vi "LV to ITX Retrieve Equation.vi"(0 "File or Folder Path":path=path "\\\\TILES\\Data/SA02777G.graphene.20150414/12 - sweep B +-2T, step Vsg", 5 "offset":i32, 7 "length":i32=10, 9 "index":T1={"a"=3, "b"=5, "c"=7, "d"=9, "f"=2, "N1"=2, "N2"=0, "N3"=0, "N4"=0, "g"=2}) -> (4 "y1 vs g":cluster{dbl[], dbl[]}[](graph), 6 "y2 vs g":cluster{dbl[], dbl[]}[](graph), 8 "2D":dbl[][](graph), 10 "N":cluster{"N1":dbl, "N2":dbl, "N3":dbl, "N4":dbl}={"N1"=0.0, "N2"=3512286493.887331, "N3"=3512286493.887331, "N4"=3512286493.887331} {"N4" format="%#_6p"; "N3" format="%#_6p"; "N2" format="%#_6p"; "N1" format="%#_6p"}, 14 "Comments":string="sweep Vsg (22): 750mV to -500mV 50mV steps\r\n\r\n\r\n\r\n\r\n\r\n\r\n\r\n\r\n\r\n\r\n\r\n\r\n\r\n\r\nB=0T to 2T to -2T to 0T, 0.0104 A/s\r\n\r\n\r\n\r\n\r\n\r\n\r\n\r\n\r\n\r\n\r\n\r\n\r\n\r\n\r\n\r\n\r\n\r\n\r\n\r\n\r\n\r\n\r\n\r\n\r\n\r\n\r\n\r\n\r\n\r\nlockin\r\n\r\n\r\n\r\n\r\n\r\n\r\n\r\n\r\n\r\n\r\n\r\n\r\n\r\n\r\n0: 1\r\n\r\n\r\n\r\n\r\n\r\n\r\n\r\n\r\n\r\n\r\n\r\n\r\n\r\n\r\n1: 3\r\n\r\n\r\n\r\n\r\n\r\n\r\n\r\n\r\n\r\n\r\n\r\n\r\n\r\n\r\n2: 4, current\r\n\r\n\r\n\r\n\r\n\r\n\r\n\r\n\r\n\r\n\r\n\r\n\r\n\r\n\r\n3: 5\r\n\r\n\r\n\r\n\r\n\r\n\r\n\r\n\r\n\r\n\r\n\r\n\r\n\r\n\r\n4: 27\r\n\r\n\r\n\r\n\r\n\r\n\r\n\r\n\r\n\r\n\r\n\r\n\r\n\r\n\r\n5: 28, current, 8mV AC\r\n\r\n\r\n\r\n\r\n\r\n\r\n\r\n\r\n\r\n\r\n\r\n\r\n\r\n\r\nappliedVsg= 0.300000\r\n\r\n\r\n\r\n\r\n\r\n\r\n\r\n\r\n\r\n\r\n\r\n\r\n\r\n\r\n")   [LabVIEW 2016, in "LVtoITX.lvclass"]
uses:
  LVtoITX.lvclass
  <vilib>/Utility/miscctls.llb/LVOffsetAndMultiplierTypeDef.ctl
  <vilib>/gmath/NI_Gmath.lvlib
panel:
  in  "2D graph:\non = y1\noff = y2":bool=TRUE
  in  "DAT header length":i32=11
  in  "data length":i32=2500
  in  "data index":i32=1400
  in  "string formula":bool caption="string formula = ON (slow, easy prototyping)\nblock diagram formula = OFF (fast, must edit block diagram to change))"
  in  "Enum":enum16{"ITX", "ITX w/ 2D", "DAT"}(ring)=enum."DAT"
  in  "formula (parameters: a,b,c,d,f)":string="y1 = (a-b)/c;\ny2 = (b-d)/c;"
  in  "D  is time?":bool
  in  "B is time?":bool
  out "time":string[][](table)=[["4/18/2015", "12:40 PM"], ["4/18/2015", "5:05 PM"], ["4/18/2015", "10:04 PM"], ["4/18/2015", "11:37 PM"], ["4/19/2015", "1:07 AM"], ["4/19/2015", "2:37 AM"], ["4/19/2015", "4:07 AM"], ["4/19/2015", "5:37 AM"], ["4/19/2015", "7:08 AM"], ["4/19/2015", "8:38 AM"]]
  in  "Use Folder Index File?":bool
  in  "Generate Folder Index File?":bool
  in  "Ez name":string="Ez name"
  in  "Ey name":string="Ey name"
  in  "Ex name":string="Ex name"
  in  "C y name":string="C y name"
  in  "D x name":string="D x name"
  in  "A y name":string="A y name"
  in  "B x name":string="B x name"
  out "Index, Wavenames":string[][](table)=[["0", "time"], ["1", "temp"], ["2", "Bfield"], ["3", "X0"], ["4", "Y0"], ["5", "X1"], ["6", "Y1"], ["7", "X2"], ["8", "Y2"], ["9", "X3"], ["10", "Y3"], ["11", "X4"], ["12", "Y4"], ["13", "X5"], ["", "Y5"]]
  in  "recolor traces?":bool=TRUE
  in  "Ex":T2={"Offset"=0.0, "Multiplier"=1.0}
  in  "Ey":T2={"Offset"=0.0, "Multiplier"=1.0}
  out "Path":path=path "\\\\TILES\\Data/SA02777G.graphene.20150414/12 - sweep B +-2T, step Vsg/SA02777G.graphene.20150414.000009.dat"
  out "counter":i32=9
  in  "pattern":string="*.dat"
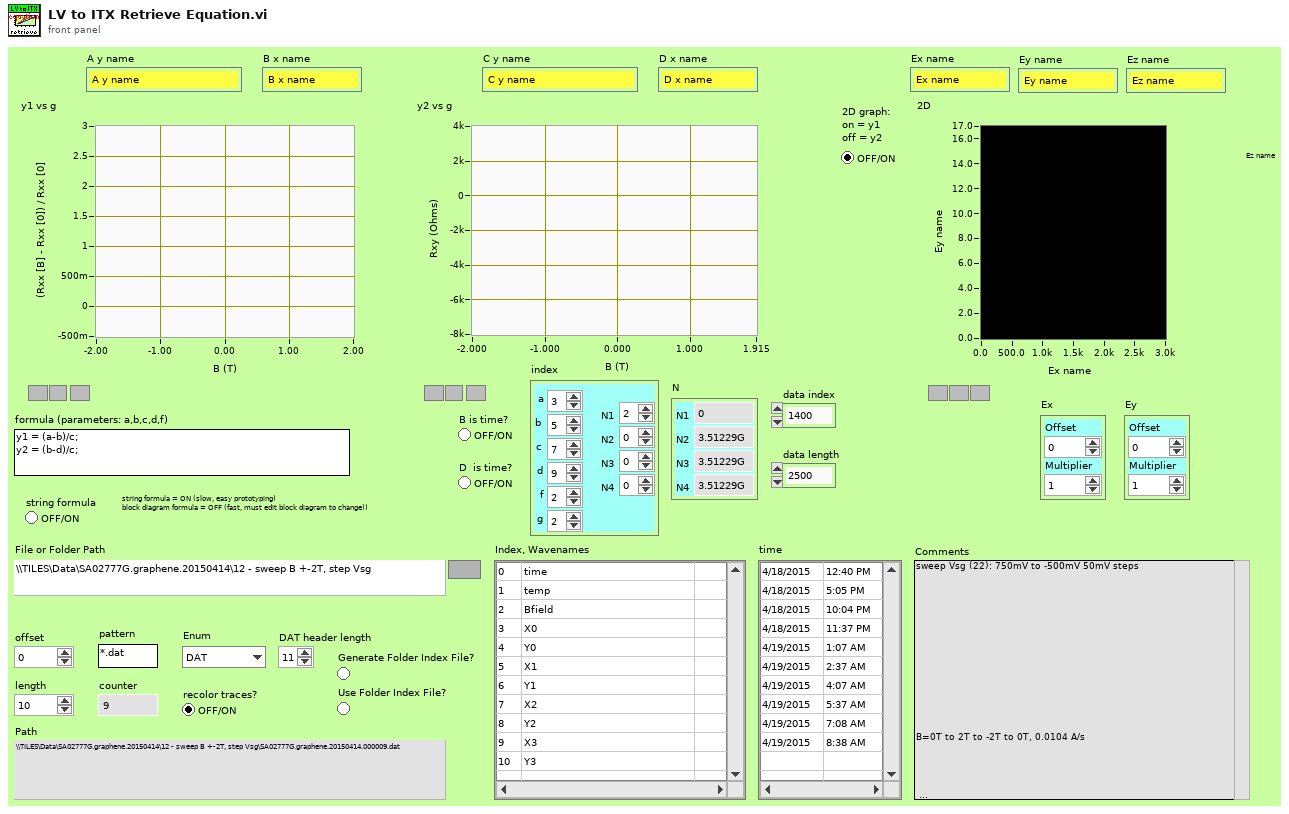
[diagram p1: front panel]
types:
  T1 = cluster{"a":i32, "b":i32, "c":i32, "d":i32, "f":i32, "N1":i32, "N2":i32, "N3":i32, "N4":i32, "g":i32}
  T2 = typedef "LVOffsetAndMultiplierTypeDef.ctl" = cluster{"Offset":dbl, "Multiplier":dbl}
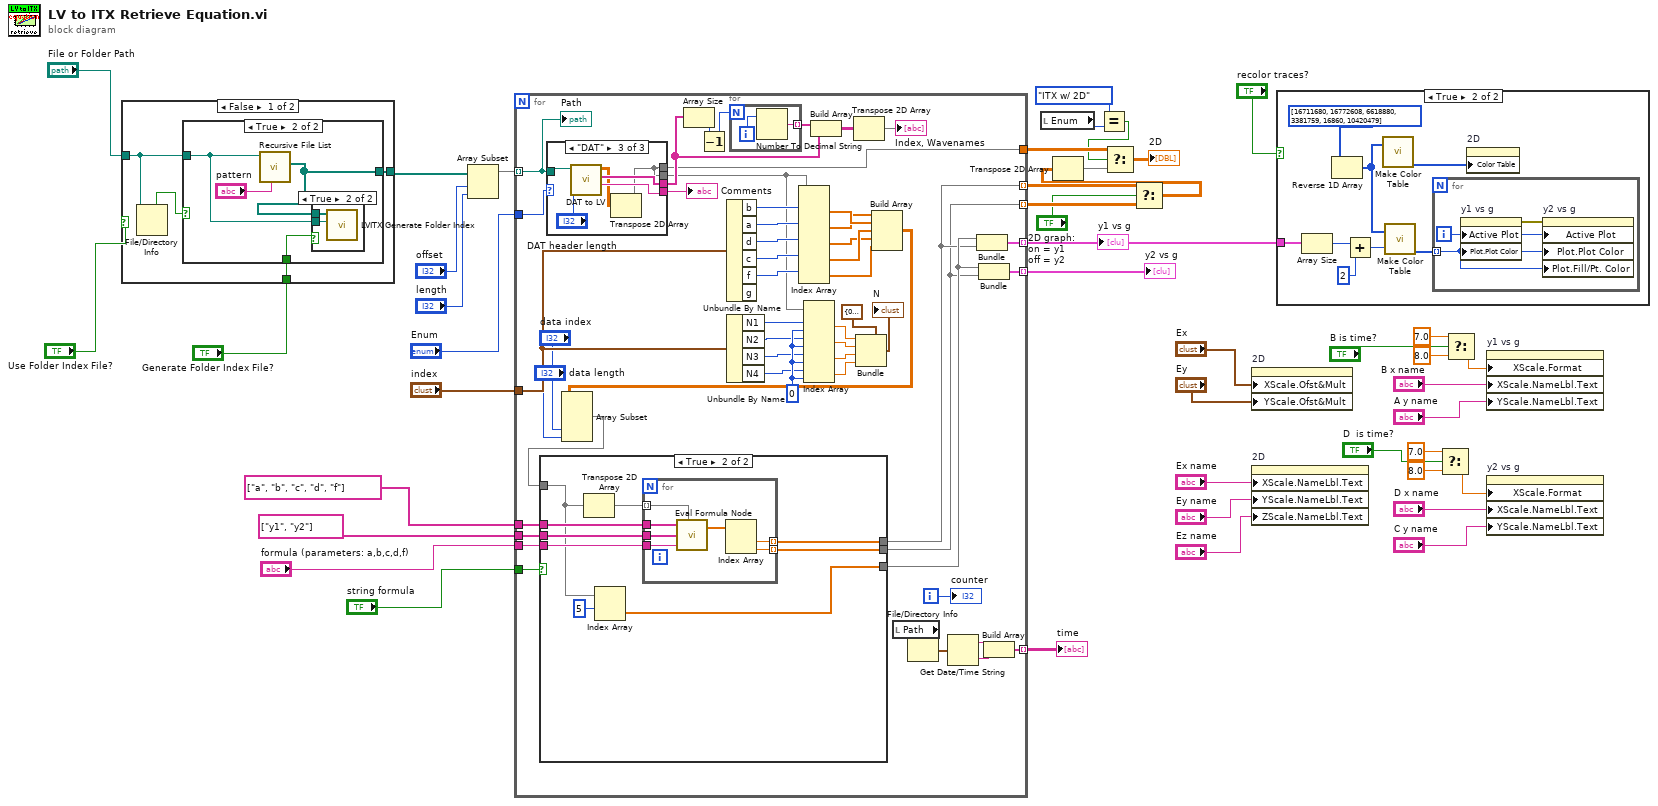
[diagram p0: block diagram]
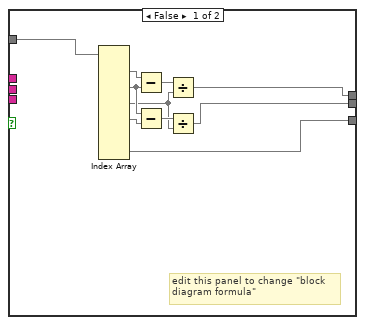
[diagram p3: hidden frame]
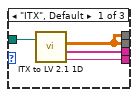
[diagram p4: hidden frame]
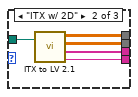
[diagram p5: hidden frame]
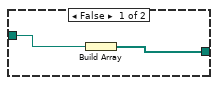
[diagram p6: hidden frame]
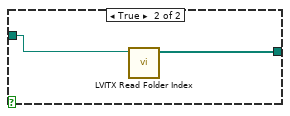
[diagram p8: hidden frame]
diagram:
  n1 = case shown="False" "Use Folder Index File?" {
    tunnel: [w46 w57] -> w42
    tunnel: "File or Folder Path" -> [w48 w58]
    tunnel: "Generate Folder Index File?" -> [w45 _]
    frame False {
      n2 = File/Directory Info(path=w48) -> (directory=w47:bool)  [unwired: 1 in, 6 out]
      n3 = case shown="True" w47 {
        tunnel: [w50 w53] -> w46
        tunnel: w48 -> [w49 w52]
        tunnel: w45 -> [_ w51]
        frame False {
          n4 = Build Array(w49) -> (w50:path[])
        }
        frame True {
          n5 = call <vilib>:"Recursive File List.vi"("pattern"="pattern", "Folder Path"=w52) -> ("All Files in Dir"=w53:path[])  [unwired: 5 in, 4 out]
          n6 = case shown="True" w51 {
            tunnel: w53 -> [_ w56]
            tunnel: w52 -> [_ w55]
            frame False {
            }
            frame True {
              n7 = call "LVITX Generate Folder Index.vi"("File or Folder Path"=w55, "All Files in Dir"=w56) -> ()  [unwired: 10 in]
            }
          }
        }
      }
    }
    frame True {
      n8 = call "LVITX Read Folder Index.vi"("File or Folder Path"=w58) -> ("Array"=w57:path[])  [unwired: 10 in]
    }
  }
  n9 = Array Subset(array=w42, index="offset", length="length") -> (w22:path[])
  n10 = for {
    tunnel: w22 -> [w108] mode=indexing
    tunnel: [w108] -> _ mode=indexing
    tunnel: [w107] -> w10 mode=indexing
    tunnel: [w106] -> w33 mode=indexing
    tunnel: [w99] -> w35
    tunnel: [w85] -> w25 mode=indexing
    tunnel: "formula (parameters: a,b,c,d,f)" -> [w74]
    tunnel: string[] ["y1", "y2"] ("Variables Output") -> [w73]
    tunnel: string[] ["a", "b", "c", "d", "f"] ("Variables Input") -> [w72]
    tunnel: "Enum" -> [w71]
    tunnel: "index" -> [w70]
    tunnel: "string formula" -> [w69]
    tunnel: [w62] -> w4 mode=indexing
    tunnel: [w61] -> w2 mode=indexing
    i -> [w110]
    w98 = 0 ("disabled index (col)")
    n11 = case shown="\"DAT\"" w71 {
      tunnel: [w142 w145 w152] -> w109
      tunnel: [w140 w146 w149] -> w75
      tunnel: w108 -> [w141 w147 w153]
      tunnel: [w139 w144 w151] -> w100
      tunnel: [w140 w143 w149] -> w99
      frame "ITX", Default {
        n12 = call "ITX to LV 2.1 1D.vi"("file (use dialog)"=w141) -> ("1D arrays"=w140:dbl[][], "wave names"=w139:string[], "Notes"=w142:string)  [unwired: 2 in]
      }
      frame "ITX w/ 2D" {
        n13 = call "ITX to LV 2.1.vi"("file (use dialog)"=w147) -> ("2D array"=w143:dbl[][], "1D arrays"=w146:dbl[][], "wave names"=w144:string[], "Notes"=w145:string)  [unwired: 1 in]
      }
      frame "DAT" {
        n14 = call "DAT to LV.vi"("header length"="DAT header length", "File Path"=w153) -> ("Comments"=w152:string, "Wavenames"=w151:string[], "Data"=w150:dbl[][])  [unwired: 7 in]
        n15 = Transpose 2D Array(2D array=w150) -> (transposed array=w149:dbl[][])
      }
    }
    "Comments" <- w109
    n16 = Array Size(array=w100) -> (size(s)=w103:i32)
    n17 = Decrement(x=w103) -> (x-1=w102:i32)
    n18 = Unbundle By Name(w70) -> ("b"=w93:i32, "a"=w92:i32, "d"=w91:i32, "c"=w90:i32, "f"=w77:i32)  [unwired: 1 out]
    n19 = Unbundle By Name(w70) -> ("N1"=w94:i32, "N2"=w95:i32, "N3"=w96:i32, "N4"=w97:i32)
    n20 = for {
      N: w102 -> [_]
      tunnel: [w137] -> w105 mode=indexing
      i -> [w138]
      n21 = Number To Decimal String(number=w138) -> (decimal integer string=w137:string)  [unwired: 1 in]
    }
    n22 = Index Array(array=w75, index (row) #1=w93, index (row) #2=w92, index (row) #3=w91, index (row) #4=w90, index (row) #5=w77) -> (element #1=w84:dbl[], element #2=w78:dbl[], element #3=w76:dbl[], element #4=w83:dbl[], element #5=w65:dbl[])  [unwired: 5 in]
    n23 = Index Array(array=w75, index (row) #1=w94, index (col) #1=w98, index (row) #2=w95, index (col) #2=w98, index (row) #3=w96, index (col) #3=w98, index (row) #4=w97, index (col) #4=w98) -> (element #1=w82:dbl, element #2=w81:dbl, element #3=w80:dbl, element #4=w79:dbl)
    n24 = Build Array(w105, w100) -> (w101:string[][])
    n25 = Transpose 2D Array(2D array=w101) -> (transposed array=→"Index, Wavenames":string[][])
    n26 = Bundle(cluster=cluster{"N1":dbl, "N2":dbl, "N3":dbl, "N4":dbl} {"N1"=0.0, "N2"=0.0, "N3"=0.0, "N4"=0.0}, "N1"=w82, "N2"=w81, "N3"=w80, "N4"=w79) -> (→"N":cluster{"N1":dbl, "N2":dbl, "N3":dbl, "N4":dbl})
    n27 = Build Array(w78, w84, w83, w76, w65) -> (w60:dbl[][])
    n28 = Array Subset(array=w60, index (col)="data index", length (col)="data length") -> (w64:dbl[][])  [unwired: 2 in]
    n29 = case shown="True" w69 {
      tunnel: [w113 w129] -> w61
      tunnel: w64 -> [w111 w123]
      tunnel: [w112 w128] -> w62
      tunnel: w74 -> [_ w127]
      tunnel: w73 -> [_ w126]
      tunnel: w72 -> [_ w125]
      tunnel: [w114 w121] -> w63
      frame False {
        # "edit this panel to change \"block\ndiagram formula\""
        n30 = Index Array(array=w111) -> (element #1=w120:dbl[], element #2=w119:dbl[], element #3=w115:dbl[], element #4=w118:dbl[], element #6=w114:dbl[])  [unwired: 12 in, 1 out]
        n31 = Subtract(x=w120, y=w119) -> (x-y=w117:dbl[])
        n32 = Subtract(x=w119, y=w118) -> (x-y=w116:dbl[])
        n33 = Divide(x=w117, y=w115) -> (x/y=w112:dbl[])
        n34 = Divide(x=w116, y=w115) -> (x/y=w113:dbl[])
      }
      frame True {
        n35 = Transpose 2D Array(2D array=w123) -> (transposed array=w124:dbl[][])
        n36 = Index Array(array=w123, index (row)=5) -> (element=w121:dbl[])  [unwired: 1 in]
        n37 = for {
          tunnel: w125 -> [w136]
          tunnel: w126 -> [w135]
          tunnel: w127 -> [w134]
          tunnel: w124 -> [w130] mode=indexing
          tunnel: [w132] -> w129 mode=indexing
          tunnel: [w131] -> w128 mode=indexing
          n38 = call <vilib>:"Eval Formula Node.vi"("Variables Input"=w136, "Input Values"=w130, "Variables Output"=w135, "formula"=w134) -> ("Output Values"=w133:dbl[])  [unwired: 1 in, 1 out]
          n39 = Index Array(array=w133) -> (element #1=w131:dbl, element #2=w132:dbl)  [unwired: 2 in]
        }
      }
    }
    n40 = local read "Path"() -> (w89:path)
    n41 = File/Directory Info(path=w89) -> (last mod=w88:timestamp)  [unwired: 1 in, 6 out]
    n42 = Get Date/Time String(seconds (now)=w88) -> (date string=w87:string, time string=w86:string)  [unwired: 2 in]
    n43 = Bundle(w63, w62) -> (w107:cluster{dbl[], dbl[]})  [unwired: 1 in]
    n44 = Bundle(w63, w61) -> (w106:cluster{dbl[], dbl[]})  [unwired: 1 in]
    n45 = Build Array(w87, w86) -> (w85:string[])
    "counter" <- w110
    "Path" <- w108
  }
  "y1 vs g" <- w10
  "y2 vs g" <- w33
  "time" <- w25
  n46 = local read "Enum"() -> (w12:enum16{"ITX", "ITX w/ 2D", "DAT"})
  n47 = Equal?(x=enum16{"ITX", "ITX w/ 2D", "DAT"}."ITX w/ 2D" ("Enum"), y=w12) -> (x = y?=w11:bool)
  n48 = Select(t=w4, s="2D graph:\non = y1\noff = y2", f=w2) -> (s? t:f=w3:dbl[][])
  n49 = Transpose 2D Array(2D array=w3) -> (transposed array=w37:dbl[][])
  n50 = Select(t=w35, s=w11, f=w37) -> (s? t:f=→"2D":dbl[][])
  n51 = property on="2D" class="IntGraph (strict)"("XScale.Ofst&Mult"="Ex", "YScale.Ofst&Mult"="Ey") -> ()  [unwired: 2 in, 2 out]
  n52 = property on="2D" class="IntGraph (strict)"("XScale.NameLbl.Text"="Ex name", "YScale.NameLbl.Text"="Ey name", "ZScale.NameLbl.Text"="Ez name") -> ()  [unwired: 2 in, 2 out]
  n53 = case shown="True" "recolor traces?" {
    tunnel: w10 -> [_ w156]
    frame False {
    }
    frame True {
      n54 = Array Size(array=w156) -> (size(s)=w157:i32)
      n55 = Reverse 1D Array(array=u32[] [16711680, 16772608, 6618880, 3381759, 16860, 10420479] ("color scale")) -> (reversed array=w155:u32[])
      n56 = Add(x=w157, y=2 ("x")) -> (x+y=w161:i32)
      n57 = call <userlib>:"Make Color Table.vi"("Array"=w155) -> ("Color Tbl"=w159:u32[])  [unwired: 1 in, 3 out]
      n58 = call <userlib>:"Make Color Table.vi"("Array"=w155, "Size/3"=w161) -> ("Color Tbl"=w158:u32[])  [unwired: 3 out]
      n59 = for {
        tunnel: w158 -> [w162] mode=indexing
        i -> [w163]
        n60 = property on="y1 vs g" class="XYGraph (strict)"("Active Plot"=w163, "Plot.Plot Color"=w162) -> (error out=w164:errorcluster)  [unwired: 2 in, 1 out]
        n61 = property on="y2 vs g" class="XYGraph (strict)"(error in=w164, "Active Plot"=w163, "Plot.Plot Color"=w162, "Plot.Fill/Pt. Color"=w162) -> ()  [unwired: 1 in, 2 out]
      }
      n62 = property on="2D" class="IntGraph (strict)"("Color Table"=w159) -> ()  [unwired: 2 in, 2 out]
    }
  }
  n63 = Select(t=7.0, s="D  is time?", f=8.0) -> (s? t:f=w18:dbl)
  n64 = Select(t=7.0, s="B is time?", f=8.0) -> (s? t:f=w19:dbl)
  n65 = property on="y1 vs g" class="XYGraph (strict)"("XScale.Format"=w19, "XScale.NameLbl.Text"="B x name", "YScale.NameLbl.Text"="A y name") -> ()  [unwired: 2 in, 2 out]
  n66 = property on="y2 vs g" class="XYGraph (strict)"("XScale.Format"=w18, "XScale.NameLbl.Text"="D x name", "YScale.NameLbl.Text"="C y name") -> ()  [unwired: 2 in, 2 out]
